vi "DCT变换优化算法.vi"(0 "模块选择簇":T3, 5 "光源散斑簇":T1, 7 "图像簇":T2) -> (4 "散斑图像作用结果":dbl[][](array[numeric]), 6 "优化光源散斑簇":T1, 8 "优化图像簇":T2)   [LabVIEW 2018]
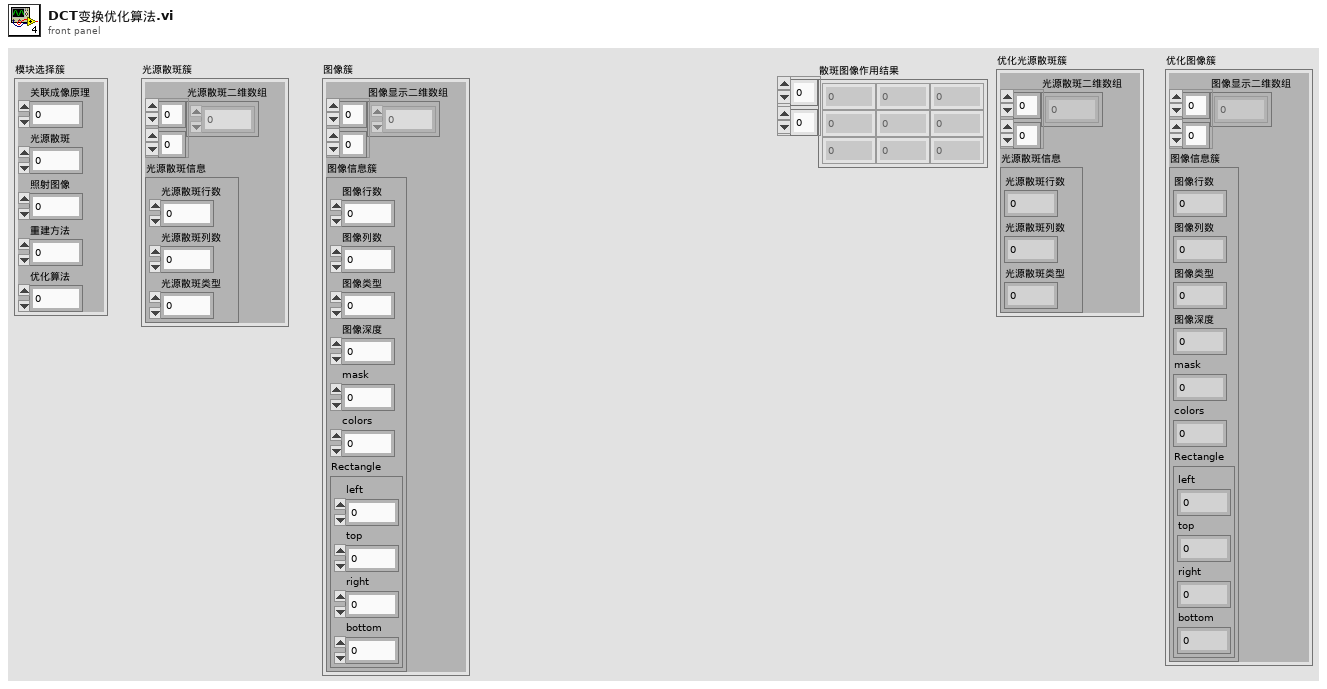
[diagram p1: front panel]
types:
  T1 = cluster{"光源散斑二维数组":dbl[][], "光源散斑信息":cluster{"光源散斑行数":dbl, "光源散斑列数":dbl, "光源散斑类型":dbl}}
  T2 = cluster{"图像显示二维数组":dbl[][], "图像信息簇":cluster{"图像行数":dbl, "图像列数":dbl, "图像类型":dbl, "图像深度":i32, "mask":i32, "colors":i32, "Rectangle":cluster{"left":i16, "top":i16, "right":i16, "bottom":i16}}}
  T3 = cluster{"关联成像原理":i32, "光源散斑":i32, "照射图像":i32, "重建方法":i32, "优化算法":i32}
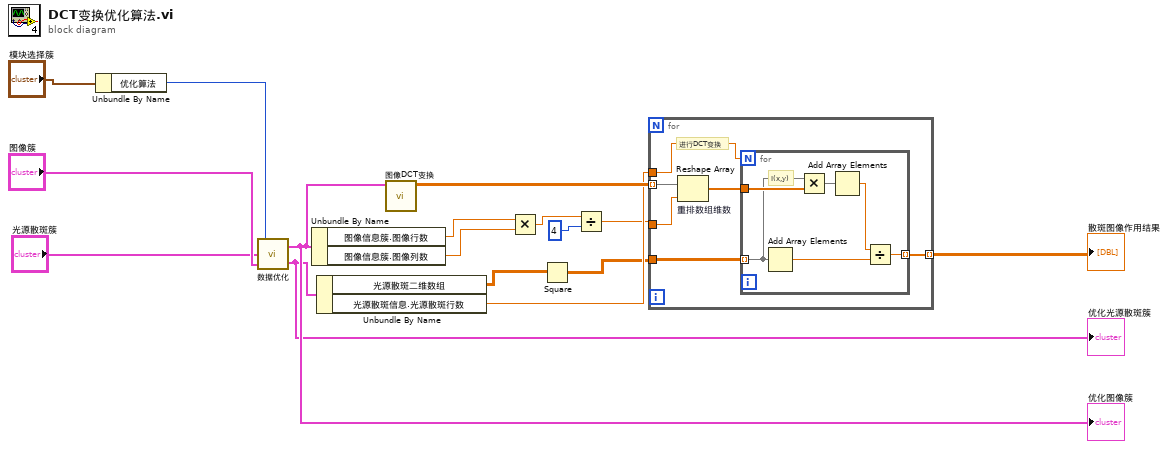
[diagram p0: block diagram]
diagram:
  n1 = Unbundle By Name("模块选择簇") -> ("优化算法"=w10:i32)
  n2 = call "数据优化.vi"("图像簇"="图像簇", "光源散斑簇"="光源散斑簇", "优化算法"=w10) -> ("优化光源散斑簇"=w6:T1, "优化图像簇"=w7:T2)
  "优化图像簇" <- w7
  "优化光源散斑簇" <- w6
  n3 = Unbundle By Name(w7) -> ("图像信息簇.图像行数"=w15:dbl, "图像信息簇.图像列数"=w14:dbl)
  n4 = Unbundle By Name(w6) -> ("光源散斑二维数组"=w2:dbl[][], "光源散斑信息.光源散斑行数"=w13:dbl)
  n5 = call "图像DCT变换.vi"("图像簇"=w7) -> ("DCT变换结果"=w16:dbl[][][])  [unwired: 10 in]
  n6 = Multiply(x=w15, y=w14) -> (x*y=w5:dbl)
  n7 = Square(x=w2) -> (x^2=w1:dbl[][])
  n8 = Divide(x=w5, y=4) -> (x/y=w3:dbl)
  n9 = for {
    tunnel: w13 -> [w21]
    tunnel: w1 -> [w19]
    tunnel: [w20] -> w12 mode=indexing
    tunnel: w16 -> [w18] mode=indexing
    tunnel: w3 -> [w17]
    # "进行DCT变换"
    n10 = Reshape Array "重排数组维数"(w18, w17) -> (w22:dbl[])
    n11 = for {
      N: w21 -> [_]
      tunnel: w22 -> [w28]
      tunnel: [w24] -> w20 mode=indexing
      tunnel: w19 -> [w23] mode=indexing
      # "I(x,y)"
      n12 = Add Array Elements(numeric array=w23) -> (sum=w25:dbl)
      n13 = Multiply(x=w23, y=w28) -> (x*y=w27:dbl[])
      n14 = Add Array Elements(numeric array=w27) -> (sum=w26:dbl)
      n15 = Divide(x=w26, y=w25) -> (x/y=w24:dbl)
    }
  }
  "散斑图像作用结果" <- w12
